vi "Read Stop Bits.vi"(8 "error in (no error)":errorcluster caption="错误输入（无错误）", 11 "Serial Master输入":refnum<class "Serial Master.lvclass">) -> (0 "error out":errorcluster caption="错误输出", 2 "Stop Bits":u16(ring)=10 items=["1.0"=10, "1.5"=15, "2.0"=20], 3 "Serial Master输出":refnum<class "Serial Master.lvclass">)   [LabVIEW 2013, in "Modbus Library - Advance.lvlib" / "Serial Master.lvclass"]
uses:
  Serial Master.lvclass
  Serial Master.lvclass/Serial Master.ctl
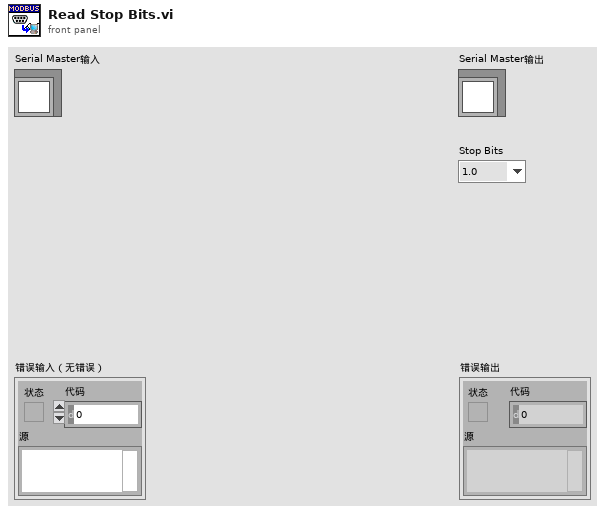
[diagram p1: front panel]
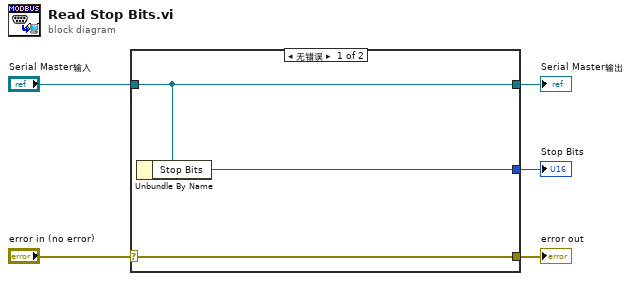
[diagram p0: block diagram]
diagram:
  n1 = case shown="无错误" "error in (no error)" {
    selector: "error in (no error)" -> [w8 w9]
    tunnel: [w8 w9] -> w4
    tunnel: [w7 w10] -> w2
    tunnel: "Serial Master输入" -> [w7 w10]
    tunnel: [w6 _] -> w1
    frame No Error {
      n2 = Unbundle By Name(w7) -> ("Stop Bits"=w6:u16)
    }
    frame Error {
    }
  }
  "error out" <- w4
  "Serial Master输出" <- w2
  "Stop Bits" <- w1
